vi "add transfer group to configuration.vi"(8 "error in (no error)":errorcluster, 9 "group info":T1, 10 "id":string, 11 "DSFConfiguration in":refnum<class "DSFConfiguration.lvclass">) -> (0 "error out":errorcluster, 3 "DSFConfiguration out":refnum<class "DSFConfiguration.lvclass">)   [LabVIEW 2017, in "DSFConfiguration.lvclass"]
uses:
  DSFConfiguration.lvclass
  IDable/IDable.lvclass
  DSFGroup/DSFGroup.lvclass
  API/1.0.0/File API/DSFConfig.lvlib
  C:/github/data-sharing-framework-custom-device/Source/Submodules/DSF/Source/Configuration API/Classes/IDable/IDable.lvclass
  Controls/dsf configuration file/1.0.0/dsf group.ctl
  Controls/dsf configuration file/1.0.0/dsf timing.ctl
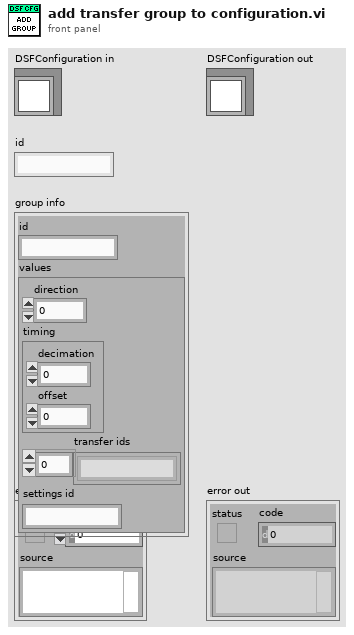
[diagram p1: front panel]
types:
  T1 = typedef "dsf configuration file v1.0.0.lvlib/dsf group.ctl" = cluster{"id":string, "values":cluster{"direction":i32, "timing":T2, "transfer ids":string[], "settings id":string}}
  T2 = typedef "dsf configuration file v1.0.0.lvlib/dsf timing.ctl" = cluster{"decimation":i32, "offset":i32}
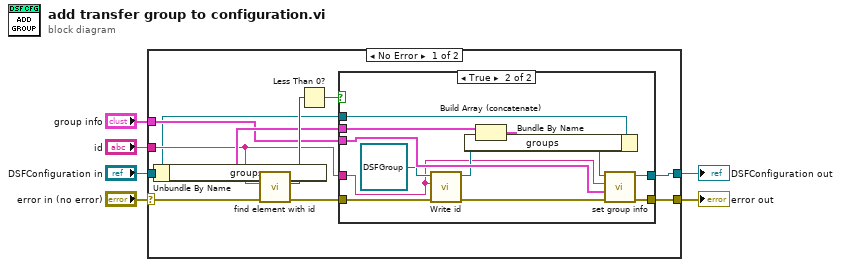
[diagram p0: block diagram]
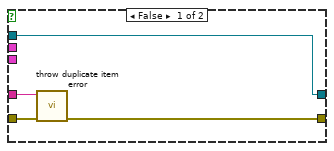
[diagram p2: hidden frame]
diagram:
  n1 = case shown="No Error" "error in (no error)" {
    selector: "error in (no error)" -> [w8 w34]
    tunnel: [w13 w34] -> w1
    tunnel: "DSFConfiguration in" -> [w9 w33]
    tunnel: "id" -> [w11 _]
    tunnel: "group info" -> [w12 _]
    tunnel: [w10 w33] -> w2
    frame No Error {
      n2 = Unbundle By Name(w9) -> ("groups"=w14:T1[])
      n3 = call "find element with id.vi"("error in (no error)"=w8, "id"=w11, "IDable Array in"=w14) -> ("error out"=w7:errorcluster, "index"=w16:i32)  [unwired: 7 in]
      n4 = Less Than 0?(x=w16) -> (x < 0?=w15:bool)
      n5 = case shown="True" w15 {
        tunnel: w14 -> [_ w32]
        tunnel: [w20 w27] -> w13
        tunnel: w7 -> [w17 w31]
        tunnel: w12 -> [_ w25]
        tunnel: w11 -> [w18 w21]
        tunnel: w9 -> [w19 w30]
        tunnel: [w19 w26] -> w10
        frame False {
          n6 = call "throw duplicate item error.vi"("error in (no error)"=w17, "id"=w18) -> ("error out"=w20:errorcluster)  [unwired: 9 in]
        }
        frame True {
          n7 = call "Write id.vi"("error in (no error)"=w31, "id"=w21, "IDable in"=refnum<class "DSFGroup.lvclass"> refnum ("DSFGroup.lvclass")) -> ("error out"=w24:errorcluster, "IDable out"=w22:refnum<class "DSFGroup.lvclass">)  [unwired: 7 in]
          n8 = Build Array (concatenate)(w32, w22) -> (w29:T1[])
          n9 = Bundle By Name(cluster=w30, "groups"=w29) -> (w28:refnum<class "DSFConfiguration.lvclass">)
          n10 = call "set group info.vi"("error in (no error)"=w24, "group info"=w25, "id"=w21, "DSFConfiguration in"=w28) -> ("error out"=w27:errorcluster, "DSFConfiguration out"=w26:refnum<class "DSFConfiguration.lvclass">)  [unwired: 6 in]
        }
      }
    }
    frame Error {
    }
  }
  "error out" <- w1
  "DSFConfiguration out" <- w2
